vi "createState.vi"(8 "error in (no error)":errorcluster, 10 "State:":T1=enum."FaultState", 11 "StateFactory in":refnum<class "StateFactory.lvclass">) -> (0 "error out":errorcluster, 2 "State.lvclass":refnum<class "State.lvclass">, 3 "StateFactory out":refnum<class "StateFactory.lvclass">)   [LabVIEW 2015, in "StateFactory.lvclass"]
uses:
  StateFactory.lvclass
  Typedefs/StateSelector.ctl
  State/State.lvclass
  States/FaultState/FaultState.lvclass
  States/OffState/OffState.lvclass
  States/StandbyState/StandbyState.lvclass
  States/EnabledState/EnabledState.lvclass
  States/WaitingForTestState/WaitingForTestState.lvclass
  States/ExecutingTestState/ExecutingTestState.lvclass
  Typedefs/ILCBTTypedefs.lvlib
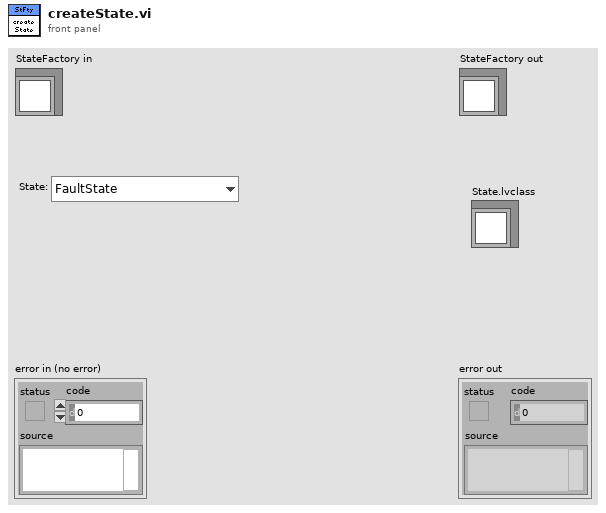
[diagram p1: front panel]
types:
  T1 = typedef "ILCBTTypedefs.lvlib/StateSelector.ctl" = enum16{"EnabledState", "FaultState", "OffState", "StandbyState", "WaitingForTestState", "ExecutingTestState"}
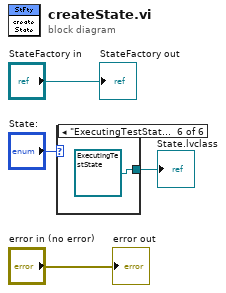
[diagram p0: block diagram]
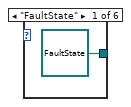
[diagram p2: hidden frame]
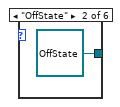
[diagram p3: hidden frame]
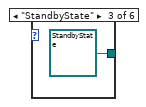
[diagram p4: hidden frame]
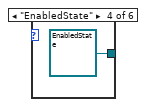
[diagram p5: hidden frame]
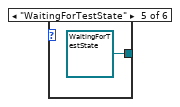
[diagram p6: hidden frame]
diagram:
  n1 = case shown="\"ExecutingTestState\"" "State:" {
    tunnel: [refnum<class "FaultState.lvclass"> refnum ("FaultState.lvclass") refnum<class "OffState.lvclass"> refnum ("ShutdownState.lvclass") refnum<class "StandbyState.lvclass"> refnum ("StandbyState.lvclass") refnum<class "EnabledState.lvclass"> refnum ("EnabledState.lvclass") refnum<class "WaitingForTestState.lvclass"> refnum ("WaitingForTestState.lvclass") refnum<class "ExecutingTestState.lvclass"> refnum ("ExecutingTestState.lvclass")] -> w1
    frame "FaultState" {
    }
    frame "OffState" {
    }
    frame "StandbyState" {
    }
    frame "EnabledState" {
    }
    frame "WaitingForTestState" {
    }
    frame "ExecutingTestState" {
    }
  }
  "State.lvclass" <- w1
  "error out" <- "error in (no error)"
  "StateFactory out" <- "StateFactory in"
